vi "Destroy.vi"(8 "error in (no error)":errorcluster, 11 "Image Undistorter in":refnum<class "Image Undistorter.lvclass">) -> (0 "error out":errorcluster)   [LabVIEW 2020, in "image.lvlib" / "Image Undistorter.lvclass"]
doc: "Destroy the Image Undistorter."
uses:
  Image Undistorter.lvclass
  Image Undistorter.lvclass/Image Undistorter.ctl
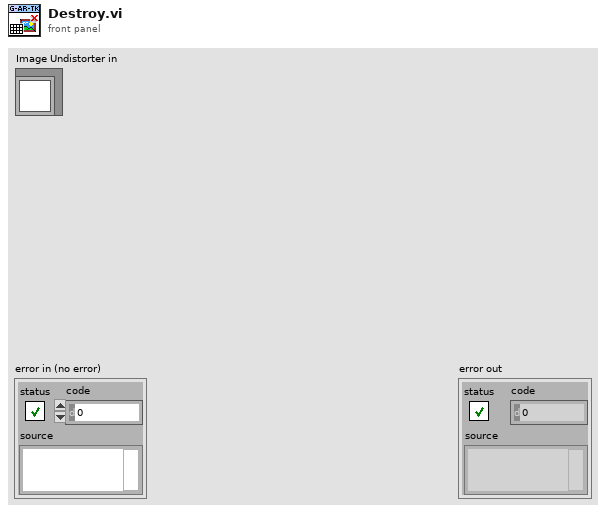
[diagram p1: front panel]
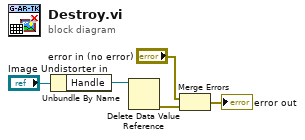
[diagram p0: block diagram]
diagram:
  n1 = Unbundle By Name("Image Undistorter in") -> ("Handle"=w3:refnum<data-value>)
  n2 = Delete Data Value Reference(data value reference=w3) -> (error out=w1:errorcluster)  [unwired: 1 in, 1 out]
  n3 = Merge Errors("error in (no error)", w1) -> (→"error out":errorcluster)
